vi "To Generic.vi"(8 "error in (no error)":errorcluster, 11 "Test Double Data in":refnum<class "Test Double Data.lvclass">) -> (0 "error out":errorcluster, 2 "Generic Data":refnum<class "Generic Data.lvclass">[](array[class]), 3 "Data Name":string[](array[string]))   [LabVIEW 2020, in "Test.lvlib" / "Test Double Data.lvclass"]
doc: "Present private data as an array of named generic data elements."
uses:
  Test Double Data.lvclass
  PPL/HDH.Data.Generic.lvlibp/Generic Data/Generic Data.lvclass
  Test Double Data.lvclass/Test Double Data.ctl
  PPL/HDH.Data.Generic.lvlibp/Generic Data/Generic Array Data/Double Array/Double Array.lvclass
  C:/Current projects/WS/PPL/HDH.Data.Generic.lvlibp/Generic Data/Generic Data.lvclass
  PPL/HDH.Actor Framework.Core.Instrument Handler.lvlibp/Data/Instrument Data/Instrument Data.lvclass
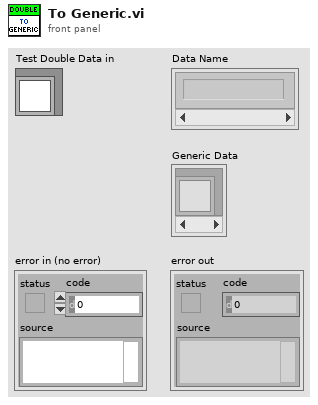
[diagram p1: front panel]
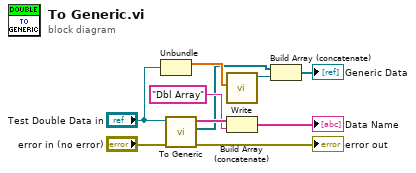
[diagram p0: block diagram]
diagram:
  n1 = Unbundle("Test Double Data in") -> (w6:dbl[])  [unwired: 1 out]
  n2 = call-parent "To Generic.vi"("error in (no error)"="error in (no error)", "Instrument Error Data in"="Test Double Data in") -> ("error out"=→"error out":errorcluster, "Generic Data"=w3:refnum<class "Generic Data.lvclass">[], "Data Name"=w9:string[])  [unwired: 7 in]
  n3 = call "Write.vi"("Double Array"=w6) -> ("Double Array out"=w1:refnum<class "Double Array.lvclass">)  [unwired: 10 in]
  n4 = Build Array (concatenate)(w9, "Dbl Array") -> (→"Data Name":string[])
  n5 = Build Array (concatenate)(w3, w1) -> (→"Generic Data":refnum<class "Generic Data.lvclass">[])
